vi "1d query test.vi"() -> ()   [LabVIEW 2020, in "mysql.lvlib" / "mysql.lvclass"]
uses:
  mysql.net/mysql.lvclass
  ed2f7c3a-0250-4def-bf4b-269ca9ba1cf2.vi
  <vilib>/Utility/error.llb/Error Cluster From Error Code.vi
panel:
  out "Result":string[](array[string])=["3.45", "10.99"]
  in  "Connection string":string="server=127.0.0.1;uid=root;pwd=Nitrog3n;database=test"
  in  "error in (no error)":errorcluster
  out "error out":errorcluster
  in  "Query string":string="SELECT price FROM shop where dealer='A';"
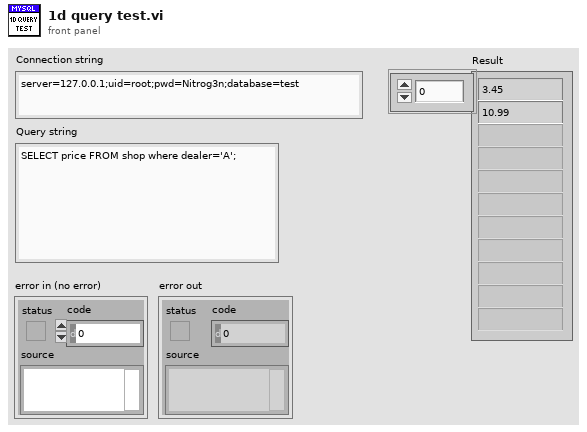
[diagram p1: front panel]
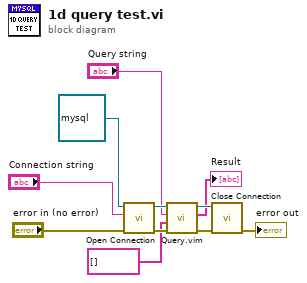
[diagram p0: block diagram]
diagram:
  n1 = call-dynamic "Open Connection.vi"("error in (no error)"="error in (no error)", "Connection string"="Connection string", "mysql in"=refnum<class "mysql.lvclass"> refnum) -> ("error out"=w10:errorcluster, "mysql out"=w11:refnum<class "mysql.lvclass">)  [unwired: 7 in]
  n2 = call "Query.vim"("error in (no error)"=w10, "Type and Default"=string[] [] ("Result 2"), "Query string"="Query string", "IDatabase in"=w11) -> ("error out"=w8:errorcluster, "Result"=→"Result":string[], "IDatabase out"=w9:refnum<class "mysql.lvclass">)  [unwired: 5 in]
  n3 = call-dynamic "Close Connection.vi"("error in (no error)"=w8, "mysql in"=w9) -> ("error out"=→"error out":errorcluster)  [unwired: 8 in, 1 out]
